vi "GetAgentClass.vi"(8 "error in":errorcluster, 10 "LibraryPath":path) -> (0 "error out":errorcluster, 1 "only one Class in Lib?":bool, 2 "Class Path":path, 5 "Class Name":string)   [LabVIEW 2009, in "HGF_VisitorGenerator.lvlib"]
doc: "Get class path from given library...\nExpected is only one class in the library...the agent class"
uses:
  HGF_VisitorGenerator.lvlib
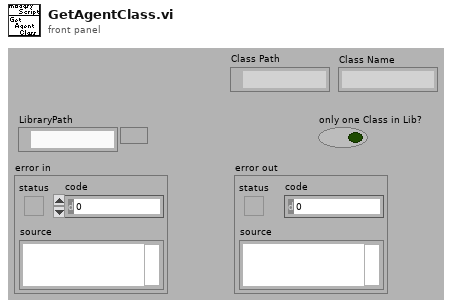
[diagram p1: front panel]
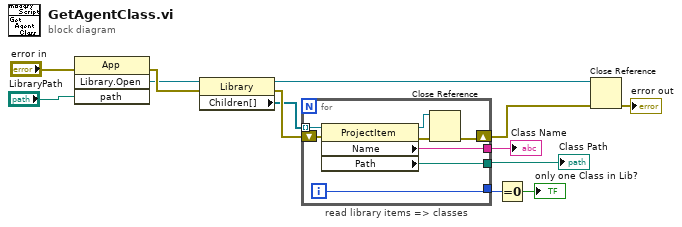
[diagram p0: block diagram]
diagram:
  n1 = invoke class="App" method="Library.Open"(error in="error in", "path"="LibraryPath") -> (error out=w7:errorcluster, "Open Library"=w6:refnum<vi>)  [unwired: 2 in, 2 out]
  n2 = property class="Library"(reference=w6, error in=w7) -> (reference out=w3:refnum<vi>, error out=w13:errorcluster, "Children[]"=w8:refnum<vi>[])
  n3 = for "read library items => classes" {
    tunnel: w8 -> [w21] mode=indexing
    tunnel: [w20] -> w10
    tunnel: [w19] -> w9
    shift-right: [w14] -> w1
    shift-left: w13 -> [w18]
    tunnel: [w17] -> w11
    i -> [w17]
    n4 = property class="ProjectItem"(reference=w21, error in=w18) -> (reference out=w16:refnum<vi>, error out=w15:errorcluster, "Name"=w20:string, "Path"=w19:path)
    n5 = Close Reference(reference=w16, error in (no error)=w15) -> (error out=w14:errorcluster)
  }
  "Class Name" <- w10
  "Class Path" <- w9
  n6 = Equal To 0?(x=w11) -> (x = 0?=→"only one Class in Lib?":bool)
  n7 = Close Reference(reference=w3, error in (no error)=w1) -> (error out=→"error out":errorcluster)
